vi "DHE_DRV_InitLib.vi"(7 "filepath":path=path "/home/bonati/panview_current/PAN/Modules/SDSU/private/c/lib/libsdsugenIII_pcix.so", 11 "error in (no error)":errorcluster) -> (8 "return value":i32, 15 "error out":errorcluster)   [LabVIEW 2016]
doc: "This VI closes the I/O interface with the instrument."
uses:
  c/lib/libarcDHE.so
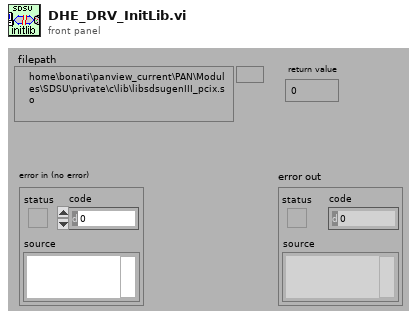
[diagram p1: front panel]
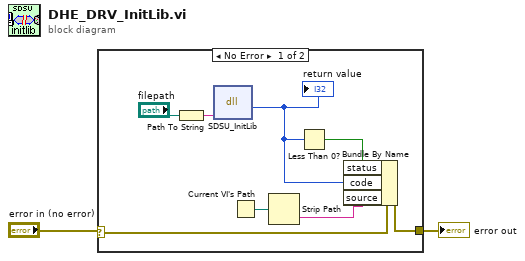
[diagram p0: block diagram]
diagram:
  n1 = case shown="No Error" "error in (no error)" {
    selector: "error in (no error)" -> [w4 w11]
    tunnel: [w6 w11] -> w2
    frame No Error {
      n2 = Path To String(path="filepath") -> (string=w3:string)
      n3 = dll-call lib="home/simager/panview/PAN/Modules/SDSU/private/c/lib/libarcDHE.so" fn="SDSU_InitLib" label="InitLib"("filepath"=w3) -> ("return type"=w9:i32)  [unwired: 4 in, 2 out]
      "return value" <- w9
      n4 = Current VI's Path() -> (path=w8:path)
      n5 = Strip Path(path=w8) -> (name=w7:string)  [unwired: 1 out]
      n6 = Less Than 0?(x=w9) -> (x < 0?=w10:bool)
      n7 = Bundle By Name(cluster=w4, "status"=w10, "code"=w9, "source"=w7) -> (w6:errorcluster)
    }
    frame Error {
    }
  }
  "error out" <- w2
